vi "输入数据解析.vi"(0 "单个参数补充":dbl, 1 "从板号":dbl=1.0, 2 "主板二维码":string="BNET01", 3 "从板二维码":string="BNET01", 5 "主板引用":refnum<vi>, 7 "从板引用":refnum<vi>, 9 "主板选项":string="三级故障阀值", 11 "枚举":enum16{"主板", "从板"}(ring), 12 "快换":bool caption="快换写入") -> (4 "输出数组":dbl[][](array[numeric]), 6 "数组长度":dbl[](array[numeric]), 8 "循环次数":i32, 10 "命令":u32, 14 "名称":string[](array[string]), 15 "命令序号":u32[](array[numeric]))   [LabVIEW 2013] (continued)
                  frame Enabled {
                    w10767 = 255 ("高字节1")
                  }
                }
                n4141 = Build Array(w10759, w10757) -> (w10758:i32[])
              }
              frame 7 {
                # "单体电压过高"
                n4142 = disable-structure shown="启用" {
                  disable-tunnel: [w10776 w10779] -> w10771
                  disable-tunnel: [w10774 w10779] -> w10769
                  disable-tunnel: w10768 -> [w10773 _]
                  frame Disabled {
                    n4143 = Unbundle By Name(w10773) -> ("单体电压过高"=w10772:dbl)
                    n4144 = call "输入分辨率计算-EV05.vi"("1字节?"=FALSE, "数值"=w10772, "偏移量"=0.0, "分辨率"=0.001) -> ("低字节"=w10774:dbl, "高字节1"=w10776:dbl)  [unwired: 1 in, 5 out]
                  }
                  frame Enabled {
                    w10779 = 255 ("高字节1")
                  }
                }
                n4145 = Build Array(w10771, w10769) -> (w10770:i32[])
              }
              frame 8 {
                # "单体电压过低"
                n4146 = disable-structure shown="启用" {
                  disable-tunnel: [w10788 w10791] -> w10783
                  disable-tunnel: [w10786 w10791] -> w10781
                  disable-tunnel: w10780 -> [w10785 _]
                  frame Disabled {
                    n4147 = Unbundle By Name(w10785) -> ("单体电压过低"=w10784:dbl)
                    n4148 = call "输入分辨率计算-EV05.vi"("1字节?"=FALSE, "数值"=w10784, "偏移量"=0.0, "分辨率"=0.001) -> ("低字节"=w10786:dbl, "高字节1"=w10788:dbl)  [unwired: 1 in, 5 out]
                  }
                  frame Enabled {
                    w10791 = 255 ("高字节1")
                  }
                }
                n4149 = Build Array(w10783, w10781) -> (w10782:i32[])
              }
              frame 9 {
                # "充电电流过高"
                n4150 = disable-structure shown="启用" {
                  disable-tunnel: [w10800 w10803] -> w10795
                  disable-tunnel: [w10798 w10803] -> w10793
                  disable-tunnel: w10792 -> [w10797 _]
                  frame Disabled {
                    n4151 = Unbundle By Name(w10797) -> ("充电电流过高"=w10796:dbl)
                    n4152 = call "输入分辨率计算-EV05.vi"("1字节?"=FALSE, "数值"=w10796, "偏移量"=-3000.0, "分辨率"=0.1) -> ("低字节"=w10798:dbl, "高字节1"=w10800:dbl)  [unwired: 1 in, 5 out]
                  }
                  frame Enabled {
                    w10803 = 255 ("高字节1")
                  }
                }
                n4153 = Build Array(w10795, w10793) -> (w10794:i32[])
              }
              frame 10 {
                # "放电电流过高"
                n4154 = disable-structure shown="启用" {
                  disable-tunnel: [w10812 w10815] -> w10807
                  disable-tunnel: [w10810 w10815] -> w10805
                  disable-tunnel: w10804 -> [w10809 _]
                  frame Disabled {
                    n4155 = Unbundle By Name(w10809) -> ("放电电流过高"=w10808:dbl)
                    n4156 = call "输入分辨率计算-EV05.vi"("1字节?"=FALSE, "数值"=w10808, "偏移量"=-3000.0, "分辨率"=0.1) -> ("低字节"=w10810:dbl, "高字节1"=w10812:dbl)  [unwired: 1 in, 5 out]
                  }
                  frame Enabled {
                    w10815 = 255 ("高字节1")
                  }
                }
                n4157 = Build Array(w10807, w10805) -> (w10806:i32[])
              }
              frame 11 {
                # "单组温度不均衡"
                n4158 = disable-structure shown="启用" {
                  disable-tunnel: [w10822 255 ("高字节1")] -> w10818
                  disable-tunnel: w10816 -> [w10820 _]
                  frame Disabled {
                    n4159 = Unbundle By Name(w10820) -> ("单组温度不均衡"=w10819:dbl)
                    n4160 = call "输入分辨率计算-EV05.vi"("1字节?"=TRUE, "数值"=w10819, "偏移量"=0.0, "分辨率"=1.0) -> ("高字节1"=w10822:dbl)  [unwired: 1 in, 6 out]
                  }
                  frame Enabled {
                  }
                }
                n4161 = Build Array(w10818) -> (w10817:i32[])
              }
              frame 12 {
                # "SOC过高"
                n4162 = Unbundle By Name(w10830) -> ("SOC过高"=w10829:dbl)
                n4163 = call "输入分辨率计算-EV05.vi"("1字节?"=FALSE, "数值"=w10829, "偏移量"=0.0, "分辨率"=0.1) -> ("低字节"=w10831:dbl, "高字节1"=w10832:dbl)  [unwired: 1 in, 5 out]
                n4164 = call "二进制解析-8.6.vi"("索引"=4, "数值"=w10832) -> ("低位子数组"=w10835:i32[])  [unwired: 3 out]
                n4165 = call "二进制解析-8.6.vi"("索引"=4, "数值"=w10831) -> ("低位子数组"=w10827:i32[], "高位子数组"=w10834:i32[])  [unwired: 2 out]
                n4166 = Insert Into Array(array=w10835, new element=w10834) -> (w10833:i32[])  [unwired: 1 in]
                n4167 = call "数值二进制转十进制-8.6.vi"("子数组"=w10833) -> ("十进制数值"=w10828:i32)  [unwired: 4 out]
                n4168 = disable-structure shown="启用" {
                  disable-tunnel: w10828 -> [w10843 _]
                  disable-tunnel: [w10843 255 ("高字节1")] -> w10826
                  disable-tunnel: w10827 -> [w10842 _]
                  disable-tunnel: [w10842 i32[] [] ("低位子数组 29")] -> _
                  frame Disabled {
                  }
                  frame Enabled {
                  }
                }
                n4169 = Build Array(w10826, w10826) -> (w10839:i32[])
              }
              frame 13 {
                # "SOC过低"
                n4170 = Unbundle By Name(w10851) -> ("SOC过低"=w10850:dbl)
                n4171 = call "输入分辨率计算-EV05.vi"("1字节?"=FALSE, "数值"=w10850, "偏移量"=0.0, "分辨率"=0.1) -> ("低字节"=w10848:dbl, "高字节1"=w10849:dbl)  [unwired: 1 in, 5 out]
                n4172 = call "二进制解析-8.6.vi"("索引"=4, "数值"=w10849) -> ("低位子数组"=w10847:i32[])  [unwired: 3 out]
                n4173 = disable-structure shown="启用" {
                  disable-tunnel: w10848 -> [w10859 _]
                  disable-tunnel: [w10859 255 ("高字节1")] -> w10846
                  disable-tunnel: [i32[] [] ("低位子数组 4") _] -> _
                  disable-tunnel: w10847 -> [w10858 _]
                  disable-tunnel: [w10858 i32[] [] ("低位子数组")] -> _
                  frame Disabled {
                  }
                  frame Enabled {
                  }
                }
                n4174 = Build Array(w10846, w10846) -> (w10854:i32[])
              }
              frame 14 {
                # "内阻过大"
                n4175 = disable-structure shown="启用" {
                  disable-tunnel: w10864 -> [w10869 _]
                  disable-tunnel: [w10865 255 ("高字节1")] -> w10862
                  frame Disabled {
                    n4176 = Unbundle By Name(w10869) -> ("内阻过大"=w10868:dbl)
                    n4177 = call "输入分辨率计算-EV05.vi"("1字节?"=TRUE, "数值"=w10868, "分辨率"=0.1) -> ("高字节1"=w10865:dbl)  [unwired: 2 in, 6 out]
                  }
                  frame Enabled {
                  }
                }
                n4178 = Build Array(w10862) -> (w10863:i32[])
              }
              frame 15 {
                # "极柱温度过高"
                n4179 = disable-structure shown="启用" {
                  disable-tunnel: w10873 -> [w10879 _]
                  disable-tunnel: [w10875 255 ("高字节1")] -> w10871
                  frame Disabled {
                    n4180 = Unbundle By Name(w10879) -> ("极柱温度过高"=w10878:dbl)
                    n4181 = call "输入分辨率计算-EV05.vi"("1字节?"=TRUE, "数值"=w10878, "偏移量"=-40.0, "分辨率"=1.0) -> ("高字节1"=w10875:dbl)  [unwired: 1 in, 6 out]
                  }
                  frame Enabled {
                  }
                }
                n4182 = Build Array(w10871) -> (w10872:i32[])
              }
              frame 16 {
                # "SOH过低"
                n4183 = disable-structure shown="启用" {
                  disable-tunnel: [w10886 w10892] -> w10883
                  disable-tunnel: w10882 -> [w10888 _]
                  disable-tunnel: [w10885 w10892] -> w10881
                  frame Enabled {
                    n4184 = Unbundle By Name(w10888) -> ("SOH过低"=w10887:dbl)
                    n4185 = call "输入分辨率计算-EV05.vi"("1字节?"=FALSE, "数值"=w10887, "偏移量"=0.0, "分辨率"=0.1) -> ("低字节"=w10885:dbl, "高字节1"=w10886:dbl)  [unwired: 1 in, 5 out]
                  }
                  frame Disabled {
                    w10892 = 255 ("高字节1")
                  }
                }
                n4186 = Build Array(w10883, w10881) -> (w10884:dbl[])
              }
            }
            n4187 = Insert Into Array(array=w10688, new element=w10689) -> (w10687:dbl[])  [unwired: 1 in]
          }
          n4188 = Build Array(w10684) -> (w10683:dbl[][])
          n4189 = Build Array("一级故障阀值") -> (w10674:string[])
        }
        frame "SOH过低(2)" {
          n4190 = Unbundle By Name(w10898) -> ("一级故障 2"=w10899:refnum<vi>)
          n4191 = property class="Clust (严格)"(reference=w10899) -> ("Value"=w10897:T4)  [unwired: 1 in, 2 out]
          n4192 = for {
            N: 17 -> [_]
            tunnel: w10897 -> [w10909]
            shift-right: [w10906] -> w10903
            shift-left: dbl[] [] -> [w10907]
            i -> [w10910]
            n4193 = case shown="13" w10910 {
              tunnel: w10909 -> [w10911 w10922 w10933 w10943 w10953 w10963 w10975 w10987 w10999 w11011 w11023 w11035 w11049 w11070 w11082 w11091 w11100]
              tunnel: [w10912 w10923 w10934 w10944 w10954 w10965 w10977 w10989 w11001 w11013 w11025 w11036 w11058 w11073 w11081 w11090 w11102] -> w10908
              frame 0, Default {
                # "总电压过高"
                n4194 = disable-structure shown="启用" {
                  disable-tunnel: [w10918 w10921] -> w10914
                  disable-tunnel: [w10917 w10921] -> w10913
                  disable-tunnel: w10911 -> [w10916 _]
                  frame Disabled {
                    n4195 = Unbundle By Name(w10916) -> ("总电压过高"=w10915:dbl)
                    n4196 = call "输入分辨率计算-EV05.vi"("1字节?"=FALSE, "数值"=w10915, "分辨率"=0.1) -> ("低字节"=w10918:dbl, "高字节1"=w10917:dbl)  [unwired: 2 in, 5 out]
                  }
                  frame Enabled {
                    w10921 = 255 ("高字节1")
                  }
                }
                n4197 = Build Array(w10913, w10914) -> (w10912:i32[])
              }
              frame 1 {
                # "总电压过低"
                n4198 = disable-structure shown="启用" {
                  disable-tunnel: [w10929 w10932] -> w10925
                  disable-tunnel: [w10928 w10932] -> w10924
                  disable-tunnel: w10922 -> [w10927 _]
                  frame Disabled {
                    n4199 = Unbundle By Name(w10927) -> ("总电压过低"=w10926:dbl)
                    n4200 = call "输入分辨率计算-EV05.vi"("1字节?"=FALSE, "数值"=w10926, "分辨率"=0.1) -> ("低字节"=w10929:dbl, "高字节1"=w10928:dbl)  [unwired: 2 in, 5 out]
                  }
                  frame Enabled {
                    w10932 = 255 ("高字节1")
                  }
                }
                n4201 = Build Array(w10924, w10925) -> (w10923:i32[])
              }
              frame 2 {
                # "温度过高"
                n4202 = disable-structure shown="启用" {
                  disable-tunnel: [w10939 255 ("高字节1")] -> w10935
                  disable-tunnel: w10933 -> [w10937 _]
                  frame Disabled {
                    n4203 = Unbundle By Name(w10937) -> ("温度过高"=w10936:dbl)
                    n4204 = call "输入分辨率计算-EV05.vi"("1字节?"=TRUE, "数值"=w10936, "偏移量"=-40.0, "分辨率"=1.0) -> ("高字节1"=w10939:dbl)  [unwired: 1 in, 6 out]
                  }
                  frame Enabled {
                  }
                }
                n4205 = Build Array(w10935) -> (w10934:i32[])
              }
              frame 3 {
                # "温度过低"
                n4206 = disable-structure shown="启用" {
                  disable-tunnel: [w10949 255 ("高字节1")] -> w10945
                  disable-tunnel: w10943 -> [w10947 _]
                  frame Disabled {
                    n4207 = Unbundle By Name(w10947) -> ("温度过低"=w10946:dbl)
                    n4208 = call "输入分辨率计算-EV05.vi"("1字节?"=TRUE, "数值"=w10946, "偏移量"=-40.0, "分辨率"=1.0) -> ("高字节1"=w10949:dbl)  [unwired: 1 in, 6 out]
                  }
                  frame Enabled {
                  }
                }
                n4209 = Build Array(w10945) -> (w10944:i32[])
              }
              frame 4 {
                # "整组温度不均衡"
                n4210 = disable-structure shown="启用" {
                  disable-tunnel: [w10959 255 ("高字节1")] -> w10955
                  disable-tunnel: w10953 -> [w10957 _]
                  frame Disabled {
                    n4211 = Unbundle By Name(w10957) -> ("整组温度不均衡"=w10956:dbl)
                    n4212 = call "输入分辨率计算-EV05.vi"("1字节?"=TRUE, "数值"=w10956, "偏移量"=0.0, "分辨率"=1.0) -> ("高字节1"=w10959:dbl)  [unwired: 1 in, 6 out]
                  }
                  frame Enabled {
                  }
                }
                n4213 = Build Array(w10955) -> (w10954:i32[])
              }
              frame 5 {
                # "单组电压不均衡"
                n4214 = disable-structure shown="启用" {
                  disable-tunnel: [w10971 w10974] -> w10966
                  disable-tunnel: [w10969 w10974] -> w10964
                  disable-tunnel: w10963 -> [w10968 _]
                  frame Disabled {
                    n4215 = Unbundle By Name(w10968) -> ("单组电压不均衡"=w10967:dbl)
                    n4216 = call "输入分辨率计算-EV05.vi"("1字节?"=FALSE, "数值"=w10967, "偏移量"=0.0, "分辨率"=0.001) -> ("低字节"=w10969:dbl, "高字节1"=w10971:dbl)  [unwired: 1 in, 5 out]
                  }
                  frame Enabled {
                    w10974 = 255 ("高字节1")
                  }
                }
                n4217 = Build Array(w10966, w10964) -> (w10965:i32[])
              }
              frame 6 {
                # "整组电压不均衡"
                n4218 = disable-structure shown="启用" {
                  disable-tunnel: [w10983 w10986] -> w10978
                  disable-tunnel: [w10981 w10986] -> w10976
                  disable-tunnel: w10975 -> [w10980 _]
                  frame Disabled {
                    n4219 = Unbundle By Name(w10980) -> ("整组电压不均衡"=w10979:dbl)
                    n4220 = call "输入分辨率计算-EV05.vi"("1字节?"=FALSE, "数值"=w10979, "偏移量"=0.0, "分辨率"=0.001) -> ("低字节"=w10981:dbl, "高字节1"=w10983:dbl)  [unwired: 1 in, 5 out]
                  }
                  frame Enabled {
                    w10986 = 255 ("高字节1")
                  }
                }
                n4221 = Build Array(w10978, w10976) -> (w10977:i32[])
              }
              frame 7 {
                # "单体电压过高"
                n4222 = disable-structure shown="启用" {
                  disable-tunnel: [w10995 w10998] -> w10990
                  disable-tunnel: [w10993 w10998] -> w10988
                  disable-tunnel: w10987 -> [w10992 _]
                  frame Disabled {
                    n4223 = Unbundle By Name(w10992) -> ("单体电压过高"=w10991:dbl)
                    n4224 = call "输入分辨率计算-EV05.vi"("1字节?"=FALSE, "数值"=w10991, "偏移量"=0.0, "分辨率"=0.001) -> ("低字节"=w10993:dbl, "高字节1"=w10995:dbl)  [unwired: 1 in, 5 out]
                  }
                  frame Enabled {
                    w10998 = 255 ("高字节1")
                  }
                }
                n4225 = Build Array(w10990, w10988) -> (w10989:i32[])
              }
              frame 8 {
                # "单体电压过低"
                n4226 = disable-structure shown="启用" {
                  disable-tunnel: [w11007 w11010] -> w11002
                  disable-tunnel: [w11005 w11010] -> w11000
                  disable-tunnel: w10999 -> [w11004 _]
                  frame Disabled {
                    n4227 = Unbundle By Name(w11004) -> ("单体电压过低"=w11003:dbl)
                    n4228 = call "输入分辨率计算-EV05.vi"("1字节?"=FALSE, "数值"=w11003, "偏移量"=0.0, "分辨率"=0.001) -> ("低字节"=w11005:dbl, "高字节1"=w11007:dbl)  [unwired: 1 in, 5 out]
                  }
                  frame Enabled {
                    w11010 = 255 ("高字节1")
                  }
                }
                n4229 = Build Array(w11002, w11000) -> (w11001:i32[])
              }
              frame 9 {
                # "充电电流过高"
                n4230 = disable-structure shown="启用" {
                  disable-tunnel: [w11019 w11022] -> w11014
                  disable-tunnel: [w11017 w11022] -> w11012
                  disable-tunnel: w11011 -> [w11016 _]
                  frame Disabled {
                    n4231 = Unbundle By Name(w11016) -> ("充电电流过高"=w11015:dbl)
                    n4232 = call "输入分辨率计算-EV05.vi"("1字节?"=FALSE, "数值"=w11015, "偏移量"=-3000.0, "分辨率"=0.1) -> ("低字节"=w11017:dbl, "高字节1"=w11019:dbl)  [unwired: 1 in, 5 out]
                  }
                  frame Enabled {
                    w11022 = 255 ("高字节1")
                  }
                }
                n4233 = Build Array(w11014, w11012) -> (w11013:i32[])
              }
              frame 10 {
                # "放电电流过高"
                n4234 = disable-structure shown="启用" {
                  disable-tunnel: [w11031 w11034] -> w11026
                  disable-tunnel: [w11029 w11034] -> w11024
                  disable-tunnel: w11023 -> [w11028 _]
                  frame Disabled {
                    n4235 = Unbundle By Name(w11028) -> ("放电电流过高"=w11027:dbl)
                    n4236 = call "输入分辨率计算-EV05.vi"("1字节?"=FALSE, "数值"=w11027, "偏移量"=-3000.0, "分辨率"=0.1) -> ("低字节"=w11029:dbl, "高字节1"=w11031:dbl)  [unwired: 1 in, 5 out]
                  }
                  frame Enabled {
                    w11034 = 255 ("高字节1")
                  }
                }
                n4237 = Build Array(w11026, w11024) -> (w11025:i32[])
              }
              frame 11 {
                # "单组温度不均衡"
                n4238 = disable-structure shown="启用" {
                  disable-tunnel: [w11041 255 ("高字节1")] -> w11037
                  disable-tunnel: w11035 -> [w11039 _]
                  frame Disabled {
                    n4239 = Unbundle By Name(w11039) -> ("单组温度不均衡"=w11038:dbl)
                    n4240 = call "输入分辨率计算-EV05.vi"("1字节?"=TRUE, "数值"=w11038, "偏移量"=0.0, "分辨率"=1.0) -> ("高字节1"=w11041:dbl)  [unwired: 1 in, 6 out]
                  }
                  frame Enabled {
                  }
                }
                n4241 = Build Array(w11037) -> (w11036:i32[])
              }
              frame 12 {
                # "SOC过高"
                n4242 = Unbundle By Name(w11049) -> ("SOC过高"=w11048:dbl)
                n4243 = call "输入分辨率计算-EV05.vi"("1字节?"=FALSE, "数值"=w11048, "偏移量"=0.0, "分辨率"=0.1) -> ("低字节"=w11050:dbl, "高字节1"=w11051:dbl)  [unwired: 1 in, 5 out]
                n4244 = call "二进制解析-8.6.vi"("索引"=4, "数值"=w11051) -> ("低位子数组"=w11054:i32[])  [unwired: 3 out]
                n4245 = call "二进制解析-8.6.vi"("索引"=4, "数值"=w11050) -> ("低位子数组"=w11046:i32[], "高位子数组"=w11053:i32[])  [unwired: 2 out]
                n4246 = Insert Into Array(array=w11054, new element=w11053) -> (w11052:i32[])  [unwired: 1 in]
                n4247 = call "数值二进制转十进制-8.6.vi"("子数组"=w11052) -> ("十进制数值"=w11047:i32)  [unwired: 4 out]
                n4248 = disable-structure shown="启用" {
                  disable-tunnel: w11047 -> [w11062 _]
                  disable-tunnel: [w11062 255 ("高字节1")] -> w11045
                  disable-tunnel: w11046 -> [w11061 _]
                  disable-tunnel: [w11061 i32[] [] ("低位子数组 29")] -> _
                  frame Disabled {
                  }
                  frame Enabled {
                  }
                }
                n4249 = Build Array(w11045, w11045) -> (w11058:i32[])
              }
              frame 13 {
                # "SOC过低"
                n4250 = Unbundle By Name(w11070) -> ("SOC过低"=w11069:dbl)
                n4251 = call "输入分辨率计算-EV05.vi"("1字节?"=FALSE, "数值"=w11069, "偏移量"=0.0, "分辨率"=0.1) -> ("低字节"=w11067:dbl, "高字节1"=w11068:dbl)  [unwired: 1 in, 5 out]
                n4252 = call "二进制解析-8.6.vi"("索引"=4, "数值"=w11068) -> ("低位子数组"=w11066:i32[])  [unwired: 3 out]
                n4253 = disable-structure shown="启用" {
                  disable-tunnel: w11067 -> [w11077 _]
                  disable-tunnel: [w11077 255 ("高字节1")] -> w11065
                  disable-tunnel: w11066 -> [w11076 _]
                  disable-tunnel: [w11076 i32[] [] ("低位子数组")] -> _
                  frame Disabled {
                    (unwired) i32[] [] ("低位子数组 4")
                  }
                  frame Enabled {
                  }
                }
                n4254 = Build Array(w11065, w11065) -> (w11073:i32[])
              }
              frame 14 {
                # "内阻过大"
                n4255 = disable-structure shown="启用" {
                  disable-tunnel: w11082 -> [w11087 _]
                  disable-tunnel: [w11083 255 ("高字节1")] -> w11080
                  frame Disabled {
                    n4256 = Unbundle By Name(w11087) -> ("内阻过大"=w11086:dbl)
                    n4257 = call "输入分辨率计算-EV05.vi"("1字节?"=TRUE, "数值"=w11086, "分辨率"=0.1) -> ("高字节1"=w11083:dbl)  [unwired: 2 in, 6 out]
                  }
                  frame Enabled {
                  }
                }
                n4258 = Build Array(w11080) -> (w11081:i32[])
              }
              frame 15 {
                # "极柱温度过高"
                n4259 = disable-structure shown="启用" {
                  disable-tunnel: w11091 -> [w11097 _]
                  disable-tunnel: [w11093 255 ("高字节1")] -> w11089
                  frame Disabled {
                    n4260 = Unbundle By Name(w11097) -> ("极柱温度过高"=w11096:dbl)
                    n4261 = call "输入分辨率计算-EV05.vi"("1字节?"=TRUE, "数值"=w11096, "偏移量"=-40.0, "分辨率"=1.0) -> ("高字节1"=w11093:dbl)  [unwired: 1 in, 6 out]
                  }
                  frame Enabled {
                  }
                }
                n4262 = Build Array(w11089) -> (w11090:i32[])
              }
              frame 16 {
                # "SOH过低"
                n4263 = disable-structure shown="启用" {
                  disable-tunnel: [w11104 w11110] -> w11101
                  disable-tunnel: w11100 -> [w11106 _]
                  disable-tunnel: [w11103 w11110] -> w11099
                  frame Enabled {
                    n4264 = Unbundle By Name(w11106) -> ("SOH过低"=w11105:dbl)
                    n4265 = call "输入分辨率计算-EV05.vi"("1字节?"=FALSE, "数值"=w11105, "偏移量"=0.0, "分辨率"=0.1) -> ("低字节"=w11103:dbl, "高字节1"=w11104:dbl)  [unwired: 1 in, 5 out]
                  }
                  frame Disabled {
                    w11110 = 255 ("高字节1")
                  }
                }
                n4266 = Build Array(w11101, w11099) -> (w11102:dbl[])
              }
            }
            n4267 = Insert Into Array(array=w10907, new element=w10908) -> (w10906:dbl[])  [unwired: 1 in]
          }
          n4268 = Build Array(w10903) -> (w10902:dbl[][])
          n4269 = Build Array("二级故障阀值") -> (w10893:string[])
        }
        frame "SOH过低(3)" {
          n4270 = Unbundle By Name(w11116) -> ("一级故障 3"=w11117:refnum<vi>)
          n4271 = property class="Clust (严格)"(reference=w11117) -> ("Value"=w11115:T4)  [unwired: 1 in, 2 out]
          n4272 = for {
            N: 17 -> [_]
            tunnel: w11115 -> [w11127]
            shift-right: [w11124] -> w11121
            shift-left: dbl[] [] -> [w11125]
            i -> [w11128]
            n4273 = case shown="16" w11128 {
              tunnel: w11127 -> [w11129 w11140 w11151 w11161 w11171 w11181 w11193 w11205 w11217 w11229 w11241 w11253 w11268 w11289 w11302 w11311 w11320]
              tunnel: [w11130 w11141 w11152 w11162 w11172 w11183 w11195 w11207 w11219 w11231 w11243 w11254 w11277 w11292 w11301 w11310 w11322] -> w11126
              frame 0, Default {
                # "总电压过高"
                n4274 = disable-structure shown="启用" {
                  disable-tunnel: [w11136 w11139] -> w11132
                  disable-tunnel: [w11135 w11139] -> w11131
                  disable-tunnel: w11129 -> [w11134 _]
                  frame Disabled {
                    n4275 = Unbundle By Name(w11134) -> ("总电压过高"=w11133:dbl)
                    n4276 = call "输入分辨率计算-EV05.vi"("1字节?"=FALSE, "数值"=w11133, "分辨率"=0.1) -> ("低字节"=w11136:dbl, "高字节1"=w11135:dbl)  [unwired: 2 in, 5 out]
                  }
                  frame Enabled {
                    w11139 = 255 ("高字节1")
                  }
                }
                n4277 = Build Array(w11131, w11132) -> (w11130:i32[])
              }
              frame 1 {
                # "总电压过低"
                n4278 = disable-structure shown="启用" {
                  disable-tunnel: [w11147 w11150] -> w11143
                  disable-tunnel: [w11146 w11150] -> w11142
                  disable-tunnel: w11140 -> [w11145 _]
                  frame Disabled {
                    n4279 = Unbundle By Name(w11145) -> ("总电压过低"=w11144:dbl)
                    n4280 = call "输入分辨率计算-EV05.vi"("1字节?"=FALSE, "数值"=w11144, "分辨率"=0.1) -> ("低字节"=w11147:dbl, "高字节1"=w11146:dbl)  [unwired: 2 in, 5 out]
                  }
                  frame Enabled {
                    w11150 = 255 ("高字节1")
                  }
                }
                n4281 = Build Array(w11142, w11143) -> (w11141:i32[])
              }
              frame 2 {
                # "温度过高"
                n4282 = disable-structure shown="启用" {
                  disable-tunnel: [w11157 255 ("高字节1")] -> w11153
                  disable-tunnel: w11151 -> [w11155 _]
                  frame Disabled {
                    n4283 = Unbundle By Name(w11155) -> ("温度过高"=w11154:dbl)
                    n4284 = call "输入分辨率计算-EV05.vi"("1字节?"=TRUE, "数值"=w11154, "偏移量"=-40.0, "分辨率"=1.0) -> ("高字节1"=w11157:dbl)  [unwired: 1 in, 6 out]
                  }
                  frame Enabled {
                  }
                }
                n4285 = Build Array(w11153) -> (w11152:i32[])
              }
              frame 3 {
                # "温度过低"
                n4286 = disable-structure shown="启用" {
                  disable-tunnel: [w11167 255 ("高字节1")] -> w11163
                  disable-tunnel: w11161 -> [w11165 _]
                  frame Disabled {
                    n4287 = Unbundle By Name(w11165) -> ("温度过低"=w11164:dbl)
                    n4288 = call "输入分辨率计算-EV05.vi"("1字节?"=TRUE, "数值"=w11164, "偏移量"=-40.0, "分辨率"=1.0) -> ("高字节1"=w11167:dbl)  [unwired: 1 in, 6 out]
                  }
                  frame Enabled {
                  }
                }
                n4289 = Build Array(w11163) -> (w11162:i32[])
              }
              frame 4 {
                # "整组温度不均衡"
                n4290 = disable-structure shown="启用" {
                  disable-tunnel: [w11177 255 ("高字节1")] -> w11173
                  disable-tunnel: w11171 -> [w11175 _]
                  frame Disabled {
                    n4291 = Unbundle By Name(w11175) -> ("整组温度不均衡"=w11174:dbl)
                    n4292 = call "输入分辨率计算-EV05.vi"("1字节?"=TRUE, "数值"=w11174, "偏移量"=0.0, "分辨率"=1.0) -> ("高字节1"=w11177:dbl)  [unwired: 1 in, 6 out]
                  }
                  frame Enabled {
                  }
                }
                n4293 = Build Array(w11173) -> (w11172:i32[])
              }
              frame 5 {
                # "单组电压不均衡"
                n4294 = disable-structure shown="启用" {
                  disable-tunnel: [w11189 w11192] -> w11184
                  disable-tunnel: [w11187 w11192] -> w11182
                  disable-tunnel: w11181 -> [w11186 _]
                  frame Disabled {
                    n4295 = Unbundle By Name(w11186) -> ("单组电压不均衡"=w11185:dbl)
                    n4296 = call "输入分辨率计算-EV05.vi"("1字节?"=FALSE, "数值"=w11185, "偏移量"=0.0, "分辨率"=0.001) -> ("低字节"=w11187:dbl, "高字节1"=w11189:dbl)  [unwired: 1 in, 5 out]
                  }
                  frame Enabled {
                    w11192 = 255 ("高字节1")
                  }
                }
                n4297 = Build Array(w11184, w11182) -> (w11183:i32[])
              }
              frame 6 {
                # "整组电压不均衡"
                n4298 = disable-structure shown="启用" {
                  disable-tunnel: [w11201 w11204] -> w11196
                  disable-tunnel: [w11199 w11204] -> w11194
                  disable-tunnel: w11193 -> [w11198 _]
                  frame Disabled {
                    n4299 = Unbundle By Name(w11198) -> ("整组电压不均衡"=w11197:dbl)
                    n4300 = call "输入分辨率计算-EV05.vi"("1字节?"=FALSE, "数值"=w11197, "偏移量"=0.0, "分辨率"=0.001) -> ("低字节"=w11199:dbl, "高字节1"=w11201:dbl)  [unwired: 1 in, 5 out]
                  }
                  frame Enabled {
                    w11204 = 255 ("高字节1")
                  }
                }
                n4301 = Build Array(w11196, w11194) -> (w11195:i32[])
              }
              frame 7 {
                # "单体电压过高"
                n4302 = disable-structure shown="启用" {
                  disable-tunnel: [w11213 w11216] -> w11208
                  disable-tunnel: [w11211 w11216] -> w11206
                  disable-tunnel: w11205 -> [w11210 _]
                  frame Disabled {
                    n4303 = Unbundle By Name(w11210) -> ("单体电压过高"=w11209:dbl)
                    n4304 = call "输入分辨率计算-EV05.vi"("1字节?"=FALSE, "数值"=w11209, "偏移量"=0.0, "分辨率"=0.001) -> ("低字节"=w11211:dbl, "高字节1"=w11213:dbl)  [unwired: 1 in, 5 out]
                  }
                  frame Enabled {
                    w11216 = 255 ("高字节1")
                  }
                }
                n4305 = Build Array(w11208, w11206) -> (w11207:i32[])
              }
              frame 8 {
                # "单体电压过低"
                n4306 = disable-structure shown="启用" {
                  disable-tunnel: [w11225 w11228] -> w11220
                  disable-tunnel: [w11223 w11228] -> w11218
                  disable-tunnel: w11217 -> [w11222 _]
                  frame Disabled {
                    n4307 = Unbundle By Name(w11222) -> ("单体电压过低"=w11221:dbl)
                    n4308 = call "输入分辨率计算-EV05.vi"("1字节?"=FALSE, "数值"=w11221, "偏移量"=0.0, "分辨率"=0.001) -> ("低字节"=w11223:dbl, "高字节1"=w11225:dbl)  [unwired: 1 in, 5 out]
                  }
                  frame Enabled {
                    w11228 = 255 ("高字节1")
                  }
                }
                n4309 = Build Array(w11220, w11218) -> (w11219:i32[])
              }
              frame 9 {
                # "充电电流过高"
                n4310 = disable-structure shown="启用" {
                  disable-tunnel: [w11237 w11240] -> w11232
                  disable-tunnel: [w11235 w11240] -> w11230
                  disable-tunnel: w11229 -> [w11234 _]
                  frame Disabled {
                    n4311 = Unbundle By Name(w11234) -> ("充电电流过高"=w11233:dbl)
                    n4312 = call "输入分辨率计算-EV05.vi"("1字节?"=FALSE, "数值"=w11233, "偏移量"=-3000.0, "分辨率"=0.1) -> ("低字节"=w11235:dbl, "高字节1"=w11237:dbl)  [unwired: 1 in, 5 out]
                  }
                  frame Enabled {
                    w11240 = 255 ("高字节1")
                  }
                }
                n4313 = Build Array(w11232, w11230) -> (w11231:i32[])
              }
              frame 10 {
                # "放电电流过高"
                n4314 = disable-structure shown="启用" {
                  disable-tunnel: [w11249 w11252] -> w11244
                  disable-tunnel: [w11247 w11252] -> w11242
                  disable-tunnel: w11241 -> [w11246 _]
                  frame Disabled {
                    n4315 = Unbundle By Name(w11246) -> ("放电电流过高"=w11245:dbl)
                    n4316 = call "输入分辨率计算-EV05.vi"("1字节?"=FALSE, "数值"=w11245, "偏移量"=-3000.0, "分辨率"=0.1) -> ("低字节"=w11247:dbl, "高字节1"=w11249:dbl)  [unwired: 1 in, 5 out]
                  }
                  frame Enabled {
                    w11252 = 255 ("高字节1")
                  }
                }
                n4317 = Build Array(w11244, w11242) -> (w11243:i32[])
              }
              frame 11 {
                # "单组温度不均衡"
                n4318 = disable-structure shown="启用" {
                  disable-tunnel: [w11259 255 ("高字节1")] -> w11255
                  disable-tunnel: w11253 -> [w11257 _]
                  frame Disabled {
                    n4319 = Unbundle By Name(w11257) -> ("单组温度不均衡"=w11256:dbl)
                    n4320 = call "输入分辨率计算-EV05.vi"("1字节?"=TRUE, "数值"=w11256, "偏移量"=0.0, "分辨率"=1.0) -> ("高字节1"=w11259:dbl)  [unwired: 1 in, 6 out]
                  }
                  frame Enabled {
                  }
                }
                n4321 = Build Array(w11255) -> (w11254:i32[])
              }
              frame 12 {
                # "SOC过高"
                n4322 = Unbundle By Name(w11268) -> ("SOC过高"=w11267:dbl)
                n4323 = call "输入分辨率计算-EV05.vi"("1字节?"=FALSE, "数值"=w11267, "偏移量"=0.0, "分辨率"=0.1) -> ("低字节"=w11269:dbl, "高字节1"=w11270:dbl)  [unwired: 1 in, 5 out]
                n4324 = call "二进制解析-8.6.vi"("索引"=4, "数值"=w11270) -> ("低位子数组"=w11273:i32[])  [unwired: 3 out]
                n4325 = call "二进制解析-8.6.vi"("索引"=4, "数值"=w11269) -> ("低位子数组"=w11264:i32[], "高位子数组"=w11272:i32[])  [unwired: 2 out]
                n4326 = Insert Into Array(array=w11273, new element=w11272) -> (w11271:i32[])  [unwired: 1 in]
                n4327 = call "数值二进制转十进制-8.6.vi"("子数组"=w11271) -> ("十进制数值"=w11266:i32)  [unwired: 4 out]
                n4328 = disable-structure shown="启用" {
                  disable-tunnel: w11266 -> [w11281 _]
                  disable-tunnel: [w11281 w11282] -> w11265
                  disable-tunnel: w11264 -> [w11280 _]
                  disable-tunnel: [w11280 i32[] [] ("低位子数组 29")] -> _
                  disable-tunnel: [_ w11282] -> w11263
                  frame Disabled {
                  }
                  frame Enabled {
                    w11282 = 255 ("高字节1")
                  }
                }
                n4329 = Build Array(w11265, w11263) -> (w11277:i32[])
              }
              frame 13 {
                # "SOC过低"
                n4330 = Unbundle By Name(w11289) -> ("SOC过低"=w11288:dbl)
                n4331 = call "输入分辨率计算-EV05.vi"("1字节?"=FALSE, "数值"=w11288, "偏移量"=0.0, "分辨率"=0.1) -> ("低字节"=w11286:dbl, "高字节1"=w11287:dbl)  [unwired: 1 in, 5 out]
                n4332 = call "二进制解析-8.6.vi"("索引"=4, "数值"=w11287) -> ("低位子数组"=w11285:i32[])  [unwired: 3 out]
                n4333 = disable-structure shown="启用" {
                  disable-tunnel: w11286 -> [w11297 _]
                  disable-tunnel: [w11297 255 ("高字节1")] -> w11284
                  disable-tunnel: [i32[] [] ("低位子数组 4") _] -> _
                  disable-tunnel: w11285 -> [w11296 _]
                  disable-tunnel: [w11296 i32[] [] ("低位子数组")] -> _
                  frame Disabled {
                  }
                  frame Enabled {
                  }
                }
                n4334 = Build Array(w11284, w11284) -> (w11292:i32[])
              }
              frame 14 {
                # "内阻过大"
                n4335 = disable-structure shown="启用" {
                  disable-tunnel: w11302 -> [w11307 _]
                  disable-tunnel: [w11303 255 ("高字节1")] -> w11300
                  frame Disabled {
                    n4336 = Unbundle By Name(w11307) -> ("内阻过大"=w11306:dbl)
                    n4337 = call "输入分辨率计算-EV05.vi"("1字节?"=TRUE, "数值"=w11306, "分辨率"=0.1) -> ("高字节1"=w11303:dbl)  [unwired: 2 in, 6 out]
                  }
                  frame Enabled {
                  }
                }
                n4338 = Build Array(w11300) -> (w11301:i32[])
              }
              frame 15 {
                # "极柱温度过高"
                n4339 = disable-structure shown="启用" {
                  disable-tunnel: w11311 -> [w11317 _]
                  disable-tunnel: [w11313 255 ("高字节1")] -> w11309
                  frame Disabled {
                    n4340 = Unbundle By Name(w11317) -> ("极柱温度过高"=w11316:dbl)
                    n4341 = call "输入分辨率计算-EV05.vi"("1字节?"=TRUE, "数值"=w11316, "偏移量"=-40.0, "分辨率"=1.0) -> ("高字节1"=w11313:dbl)  [unwired: 1 in, 6 out]
                  }
                  frame Enabled {
                  }
                }
                n4342 = Build Array(w11309) -> (w11310:i32[])
              }
              frame 16 {
                # "SOH过低"
                n4343 = disable-structure shown="启用" {
                  disable-tunnel: [w11324 w11330] -> w11321
                  disable-tunnel: w11320 -> [w11326 _]
                  disable-tunnel: [w11323 w11330] -> w11319
                  frame Enabled {
                    n4344 = Unbundle By Name(w11326) -> ("SOH过低"=w11325:dbl)
                    n4345 = call "输入分辨率计算-EV05.vi"("1字节?"=FALSE, "数值"=w11325, "偏移量"=0.0, "分辨率"=0.1) -> ("低字节"=w11323:dbl, "高字节1"=w11324:dbl)  [unwired: 1 in, 5 out]
                  }
                  frame Disabled {
                    w11330 = 255 ("高字节1")
                  }
                }
                n4346 = Build Array(w11321, w11319) -> (w11322:dbl[])
              }
            }
            n4347 = Insert Into Array(array=w11125, new element=w11126) -> (w11124:dbl[])  [unwired: 1 in]
          }
          n4348 = Build Array(w11121) -> (w11120:dbl[][])
          n4349 = Build Array("三级故障阀值") -> (w11111:string[])
        }
        frame "SOC过高" {
          n4350 = Unbundle By Name(w11336) -> ("一级故障"=w11337:refnum<vi>)
          n4351 = property class="Clust (严格)"(reference=w11337) -> ("Value"=w11335:T4)  [unwired: 1 in, 2 out]
          n4352 = for {
            N: 17 -> [_]
            tunnel: w11335 -> [w11347]
            shift-right: [w11344] -> w11341
            shift-left: dbl[] [] -> [w11345]
            i -> [w11348]
            n4353 = case shown="14" w11348 {
              tunnel: w11347 -> [w11349 w11360 w11371 w11381 w11391 w11401 w11413 w11425 w11437 w11449 w11461 w11473 w11486 w11493 w11505 w11514 w11523]
              tunnel: [w11350 w11361 w11372 w11382 w11392 w11403 w11415 w11427 w11439 w11451 w11463 w11474 w11488 w11494 w11504 w11513 w11525] -> w11346
              frame 0, Default {
                # "总电压过高"
                n4354 = disable-structure shown="启用" {
                  disable-tunnel: [w11356 w11359] -> w11352
                  disable-tunnel: [w11355 w11359] -> w11351
                  disable-tunnel: w11349 -> [w11354 _]
                  frame Disabled {
                    n4355 = Unbundle By Name(w11354) -> ("总电压过高"=w11353:dbl)
                    n4356 = call "输入分辨率计算-EV05.vi"("1字节?"=FALSE, "数值"=w11353, "分辨率"=0.1) -> ("低字节"=w11356:dbl, "高字节1"=w11355:dbl)  [unwired: 2 in, 5 out]
                  }
                  frame Enabled {
                    w11359 = 255 ("高字节1")
                  }
                }
                n4357 = Build Array(w11351, w11352) -> (w11350:i32[])
              }
              frame 1 {
                # "总电压过低"
                n4358 = disable-structure shown="启用" {
                  disable-tunnel: [w11367 w11370] -> w11363
                  disable-tunnel: [w11366 w11370] -> w11362
                  disable-tunnel: w11360 -> [w11365 _]
                  frame Disabled {
                    n4359 = Unbundle By Name(w11365) -> ("总电压过低"=w11364:dbl)
                    n4360 = call "输入分辨率计算-EV05.vi"("1字节?"=FALSE, "数值"=w11364, "分辨率"=0.1) -> ("低字节"=w11367:dbl, "高字节1"=w11366:dbl)  [unwired: 2 in, 5 out]
                  }
                  frame Enabled {
                    w11370 = 255 ("高字节1")
                  }
                }
                n4361 = Build Array(w11362, w11363) -> (w11361:i32[])
              }
              frame 2 {
                # "温度过高"
                n4362 = disable-structure shown="启用" {
                  disable-tunnel: [w11377 255 ("高字节1")] -> w11373
                  disable-tunnel: w11371 -> [w11375 _]
                  frame Disabled {
                    n4363 = Unbundle By Name(w11375) -> ("温度过高"=w11374:dbl)
                    n4364 = call "输入分辨率计算-EV05.vi"("1字节?"=TRUE, "数值"=w11374, "偏移量"=-40.0, "分辨率"=1.0) -> ("高字节1"=w11377:dbl)  [unwired: 1 in, 6 out]
                  }
                  frame Enabled {
                  }
                }
                n4365 = Build Array(w11373) -> (w11372:i32[])
              }
              frame 3 {
                # "温度过低"
                n4366 = disable-structure shown="启用" {
                  disable-tunnel: [w11387 255 ("高字节1")] -> w11383
                  disable-tunnel: w11381 -> [w11385 _]
                  frame Disabled {
                    n4367 = Unbundle By Name(w11385) -> ("温度过低"=w11384:dbl)
                    n4368 = call "输入分辨率计算-EV05.vi"("1字节?"=TRUE, "数值"=w11384, "偏移量"=-40.0, "分辨率"=1.0) -> ("高字节1"=w11387:dbl)  [unwired: 1 in, 6 out]
                  }
                  frame Enabled {
                  }
                }
                n4369 = Build Array(w11383) -> (w11382:i32[])
              }
              frame 4 {
                # "整组温度不均衡"
                n4370 = disable-structure shown="启用" {
                  disable-tunnel: [w11397 255 ("高字节1")] -> w11393
                  disable-tunnel: w11391 -> [w11395 _]
                  frame Disabled {
                    n4371 = Unbundle By Name(w11395) -> ("整组温度不均衡"=w11394:dbl)
                    n4372 = call "输入分辨率计算-EV05.vi"("1字节?"=TRUE, "数值"=w11394, "偏移量"=0.0, "分辨率"=1.0) -> ("高字节1"=w11397:dbl)  [unwired: 1 in, 6 out]
                  }
                  frame Enabled {
                  }
                }
                n4373 = Build Array(w11393) -> (w11392:i32[])
              }
              frame 5 {
                # "单组电压不均衡"
                n4374 = disable-structure shown="启用" {
                  disable-tunnel: [w11409 w11412] -> w11404
                  disable-tunnel: [w11407 w11412] -> w11402
                  disable-tunnel: w11401 -> [w11406 _]
                  frame Disabled {
                    n4375 = Unbundle By Name(w11406) -> ("单组电压不均衡"=w11405:dbl)
                    n4376 = call "输入分辨率计算-EV05.vi"("1字节?"=FALSE, "数值"=w11405, "偏移量"=0.0, "分辨率"=0.001) -> ("低字节"=w11407:dbl, "高字节1"=w11409:dbl)  [unwired: 1 in, 5 out]
                  }
                  frame Enabled {
                    w11412 = 255 ("高字节1")
                  }
                }
                n4377 = Build Array(w11404, w11402) -> (w11403:i32[])
              }
              frame 6 {
                # "整组电压不均衡"
                n4378 = disable-structure shown="启用" {
                  disable-tunnel: [w11421 w11424] -> w11416
                  disable-tunnel: [w11419 w11424] -> w11414
                  disable-tunnel: w11413 -> [w11418 _]
                  frame Disabled {
                    n4379 = Unbundle By Name(w11418) -> ("整组电压不均衡"=w11417:dbl)
                    n4380 = call "输入分辨率计算-EV05.vi"("1字节?"=FALSE, "数值"=w11417, "偏移量"=0.0, "分辨率"=0.001) -> ("低字节"=w11419:dbl, "高字节1"=w11421:dbl)  [unwired: 1 in, 5 out]
                  }
                  frame Enabled {
                    w11424 = 255 ("高字节1")
                  }
                }
                n4381 = Build Array(w11416, w11414) -> (w11415:i32[])
              }
              frame 7 {
                # "单体电压过高"
                n4382 = disable-structure shown="启用" {
                  disable-tunnel: [w11433 w11436] -> w11428
                  disable-tunnel: [w11431 w11436] -> w11426
                  disable-tunnel: w11425 -> [w11430 _]
                  frame Disabled {
                    n4383 = Unbundle By Name(w11430) -> ("单体电压过高"=w11429:dbl)
                    n4384 = call "输入分辨率计算-EV05.vi"("1字节?"=FALSE, "数值"=w11429, "偏移量"=0.0, "分辨率"=0.001) -> ("低字节"=w11431:dbl, "高字节1"=w11433:dbl)  [unwired: 1 in, 5 out]
                  }
                  frame Enabled {
                    w11436 = 255 ("高字节1")
                  }
                }
                n4385 = Build Array(w11428, w11426) -> (w11427:i32[])
              }
              frame 8 {
                # "单体电压过低"
                n4386 = disable-structure shown="启用" {
                  disable-tunnel: [w11445 w11448] -> w11440
                  disable-tunnel: [w11443 w11448] -> w11438
                  disable-tunnel: w11437 -> [w11442 _]
                  frame Disabled {
                    n4387 = Unbundle By Name(w11442) -> ("单体电压过低"=w11441:dbl)
                    n4388 = call "输入分辨率计算-EV05.vi"("1字节?"=FALSE, "数值"=w11441, "偏移量"=0.0, "分辨率"=0.001) -> ("低字节"=w11443:dbl, "高字节1"=w11445:dbl)  [unwired: 1 in, 5 out]
                  }
                  frame Enabled {
                    w11448 = 255 ("高字节1")
                  }
                }
                n4389 = Build Array(w11440, w11438) -> (w11439:i32[])
              }
              frame 9 {
                # "充电电流过高"
                n4390 = disable-structure shown="启用" {
                  disable-tunnel: [w11457 w11460] -> w11452
                  disable-tunnel: [w11455 w11460] -> w11450
                  disable-tunnel: w11449 -> [w11454 _]
                  frame Disabled {
                    n4391 = Unbundle By Name(w11454) -> ("充电电流过高"=w11453:dbl)
                    n4392 = call "输入分辨率计算-EV05.vi"("1字节?"=FALSE, "数值"=w11453, "偏移量"=-3000.0, "分辨率"=0.1) -> ("低字节"=w11455:dbl, "高字节1"=w11457:dbl)  [unwired: 1 in, 5 out]
                  }
                  frame Enabled {
                    w11460 = 255 ("高字节1")
                  }
                }
                n4393 = Build Array(w11452, w11450) -> (w11451:i32[])
              }
              frame 10 {
                # "放电电流过高"
                n4394 = disable-structure shown="启用" {
                  disable-tunnel: [w11469 w11472] -> w11464
                  disable-tunnel: [w11467 w11472] -> w11462
                  disable-tunnel: w11461 -> [w11466 _]
                  frame Disabled {
                    n4395 = Unbundle By Name(w11466) -> ("放电电流过高"=w11465:dbl)
                    n4396 = call "输入分辨率计算-EV05.vi"("1字节?"=FALSE, "数值"=w11465, "偏移量"=-3000.0, "分辨率"=0.1) -> ("低字节"=w11467:dbl, "高字节1"=w11469:dbl)  [unwired: 1 in, 5 out]
                  }
                  frame Enabled {
                    w11472 = 255 ("高字节1")
                  }
                }
                n4397 = Build Array(w11464, w11462) -> (w11463:i32[])
              }
              frame 11 {
                # "单组温度不均衡"
                n4398 = disable-structure shown="启用" {
                  disable-tunnel: [w11479 255 ("高字节1")] -> w11475
                  disable-tunnel: w11473 -> [w11477 _]
                  frame Disabled {
                    n4399 = Unbundle By Name(w11477) -> ("单组温度不均衡"=w11476:dbl)
                    n4400 = call "输入分辨率计算-EV05.vi"("1字节?"=TRUE, "数值"=w11476, "偏移量"=0.0, "分辨率"=1.0) -> ("高字节1"=w11479:dbl)  [unwired: 1 in, 6 out]
                  }
                  frame Enabled {
                  }
                }
                n4401 = Build Array(w11475) -> (w11474:i32[])
              }
              frame 12 {
                # "SOC过高"
                n4402 = Unbundle By Name(w11486) -> ("SOC过高"=w11485:dbl)
                n4403 = call "输入分辨率计算-EV05.vi"("1字节?"=FALSE, "数值"=w11485, "偏移量"=0.0, "分辨率"=0.1) -> ("低字节"=w11483:dbl, "高字节1"=w11484:dbl)  [unwired: 1 in, 5 out]
                n4404 = Build Array(w11484, w11483) -> (w11488:dbl[])
              }
              frame 13 {
                n4405 = disable-structure shown="启用" {
                  disable-tunnel: w11493 -> [w11498 _]
                  disable-tunnel: [w11496 w11502] -> w11492
                  disable-tunnel: [w11495 w11502] -> w11491
                  frame Disabled {
                    n4406 = Unbundle By Name(w11498) -> ("SOC过低"=w11497:dbl)
                    n4407 = call "输入分辨率计算-EV05.vi"("1字节?"=FALSE, "数值"=w11497, "偏移量"=0.0, "分辨率"=0.1) -> ("低字节"=w11495:dbl, "高字节1"=w11496:dbl)  [unwired: 1 in, 5 out]
                  }
                  frame Enabled {
                    w11502 = 255 ("高字节1")
                  }
                }
                n4408 = Build Array(w11492, w11491) -> (w11494:i32[])
              }
              frame 14 {
                # "内阻过大"
                n4409 = disable-structure shown="启用" {
                  disable-tunnel: w11505 -> [w11510 _]
                  disable-tunnel: [w11506 255 ("高字节1")] -> w11503
                  frame Disabled {
                    n4410 = Unbundle By Name(w11510) -> ("内阻过大"=w11509:dbl)
                    n4411 = call "输入分辨率计算-EV05.vi"("1字节?"=TRUE, "数值"=w11509, "分辨率"=0.1) -> ("高字节1"=w11506:dbl)  [unwired: 2 in, 6 out]
                  }
                  frame Enabled {
                  }
                }
                n4412 = Build Array(w11503) -> (w11504:i32[])
              }
              frame 15 {
                # "极柱温度过高"
                n4413 = disable-structure shown="启用" {
                  disable-tunnel: w11514 -> [w11520 _]
                  disable-tunnel: [w11516 255 ("高字节1")] -> w11512
                  frame Disabled {
                    n4414 = Unbundle By Name(w11520) -> ("极柱温度过高"=w11519:dbl)
                    n4415 = call "输入分辨率计算-EV05.vi"("1字节?"=TRUE, "数值"=w11519, "偏移量"=-40.0, "分辨率"=1.0) -> ("高字节1"=w11516:dbl)  [unwired: 1 in, 6 out]
                  }
                  frame Enabled {
                  }
                }
                n4416 = Build Array(w11512) -> (w11513:i32[])
              }
              frame 16 {
                # "SOH过低"
                n4417 = disable-structure shown="启用" {
                  disable-tunnel: [w11537 w11545] -> w11524
                  disable-tunnel: w11523 -> [w11534 _]
                  disable-tunnel: [w11526 w11545] -> w11522
                  frame Disabled {
                    n4418 = Unbundle By Name(w11534) -> ("SOH过低"=w11533:dbl)
                    n4419 = call "输入分辨率计算-EV05.vi"("1字节?"=FALSE, "数值"=w11533, "偏移量"=0.0, "分辨率"=0.1) -> ("低字节"=w11535:dbl, "高字节1"=w11536:dbl)  [unwired: 1 in, 5 out]
                    n4420 = call "二进制解析-8.6.vi"("索引"=4, "数值"=w11536) -> ("低位子数组"=w11539:i32[])  [unwired: 3 out]
                    n4421 = call "二进制解析-8.6.vi"("索引"=4, "数值"=w11535) -> ("低位子数组"=w11528:i32[], "高位子数组"=w11538:i32[])  [unwired: 2 out]
                    n4422 = call "二进制解析-8.6.vi"("索引"=4, "数值"=0) -> ("低位子数组"=w11529:i32[])  [unwired: 3 out]
                    n4423 = Insert Into Array(array=w11539, new element=w11538) -> (w11532:i32[])  [unwired: 1 in]
                    n4424 = Insert Into Array(array=w11528, new element=w11529) -> (w11527:i32[])  [unwired: 1 in]
                    n4425 = call "数值二进制转十进制-8.6.vi"("子数组"=w11532) -> ("十进制数值"=w11537:i32)  [unwired: 4 out]
                    n4426 = call "数值二进制转十进制-8.6.vi"("子数组"=w11527) -> ("十进制数值"=w11526:i32)  [unwired: 4 out]
                  }
                  frame Enabled {
                    w11545 = 255 ("高字节1")
                  }
                }
                n4427 = Build Array(w11524, w11522) -> (w11525:i32[])
              }
            }
            n4428 = Insert Into Array(array=w11345, new element=w11346) -> (w11344:dbl[])  [unwired: 1 in]
          }
          n4429 = Build Array(w11341) -> (w11340:dbl[][])
          n4430 = Build Array("一级故障阀值") -> (w11331:string[])
        }
        frame "SOC过高(2)" {
          n4431 = Unbundle By Name(w11551) -> ("一级故障 2"=w11552:refnum<vi>)
          n4432 = property class="Clust (严格)"(reference=w11552) -> ("Value"=w11550:T4)  [unwired: 1 in, 2 out]
          n4433 = for {
            N: 17 -> [_]
            tunnel: w11550 -> [w11562]
            shift-right: [w11559] -> w11556
            shift-left: dbl[] [] -> [w11560]
            i -> [w11563]
            n4434 = case shown="12" w11563 {
              tunnel: w11562 -> [w11564 w11575 w11586 w11596 w11606 w11616 w11628 w11640 w11652 w11664 w11676 w11688 w11701 w11708 w11720 w11729 w11738]
              tunnel: [w11565 w11576 w11587 w11597 w11607 w11618 w11630 w11642 w11654 w11666 w11678 w11689 w11703 w11709 w11719 w11728 w11740] -> w11561
              frame 0, Default {
                # "总电压过高"
                n4435 = disable-structure shown="启用" {
                  disable-tunnel: [w11571 w11574] -> w11567
                  disable-tunnel: [w11570 w11574] -> w11566
                  disable-tunnel: w11564 -> [w11569 _]
                  frame Disabled {
                    n4436 = Unbundle By Name(w11569) -> ("总电压过高"=w11568:dbl)
                    n4437 = call "输入分辨率计算-EV05.vi"("1字节?"=FALSE, "数值"=w11568, "分辨率"=0.1) -> ("低字节"=w11571:dbl, "高字节1"=w11570:dbl)  [unwired: 2 in, 5 out]
                  }
                  frame Enabled {
                    w11574 = 255 ("高字节1")
                  }
                }
                n4438 = Build Array(w11566, w11567) -> (w11565:i32[])
              }
              frame 1 {
                # "总电压过低"
                n4439 = disable-structure shown="启用" {
                  disable-tunnel: [w11582 w11585] -> w11578
                  disable-tunnel: [w11581 w11585] -> w11577
                  disable-tunnel: w11575 -> [w11580 _]
                  frame Disabled {
                    n4440 = Unbundle By Name(w11580) -> ("总电压过低"=w11579:dbl)
                    n4441 = call "输入分辨率计算-EV05.vi"("1字节?"=FALSE, "数值"=w11579, "分辨率"=0.1) -> ("低字节"=w11582:dbl, "高字节1"=w11581:dbl)  [unwired: 2 in, 5 out]
